vi "Write output PID.vi"(10 "output":dbl format="%.2f", 11 "PID in":refnum<class "PID.lvclass">) -> (3 "PID out":refnum<class "PID.lvclass">)   [LabVIEW 2019, in "control.lvlib" / "PID.lvclass"]
uses:
  PID.lvclass
  PID.lvclass/PID.ctl
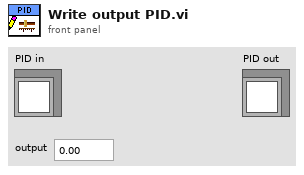
[diagram p1: front panel]
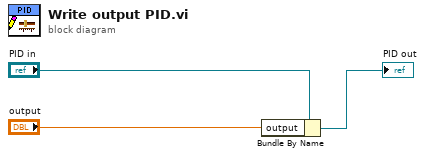
[diagram p0: block diagram]
diagram:
  n1 = Bundle By Name(cluster="PID in", "output"="output") -> (→"PID out":refnum<class "PID.lvclass">)
